vi "Save QOI Image (Path).vi"(8 "error in (no error)":errorcluster, 10 "Image":T1, 11 "Path In":path) -> (0 "error out":errorcluster, 3 "Path Out":path)   [LabVIEW 2020, in "G-Image.lvlib"]
doc: "Saves an image in QOI format to disk."
uses:
  G-Image.lvlib
  <vilib>/picture/picture.llb/imagedata.ctl
  Controls/Image Save Format.ctl
  606af2f9-acf7-4e66-8239-29e2db6da06f.vi
  Private/Debug Path.vi
  Private/Result To Error.vi
  Private/Get Image Data.vi
  Private/ARGB To RGBA.vi
  Private/Depth To Number Channels.vi
  Image Processing/Indexed Color To True Color Image.vi
  <vilib>/Utility/file.llb/Application Directory.vi
  <vilib>/Utility/error.llb/Error Cluster From Error Code.vi
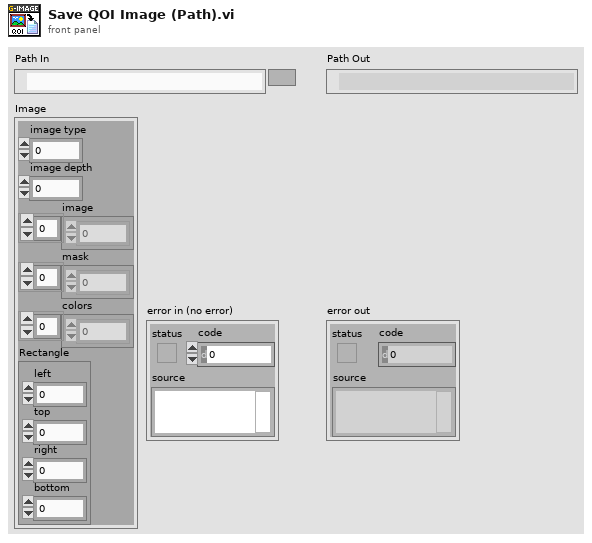
[diagram p1: front panel]
types:
  T1 = typedef "imagedata.ctl" = cluster{"image type":i32, "image depth":i32, "image":u8[], "mask":u8[], "colors":u32[], "Rectangle":cluster{"left":i16, "top":i16, "right":i16, "bottom":i16}}
  T2 = typedef "G-Image.lvlib/Image Save Format.ctl" = enum16{"png", "jpg", "bmp", "gif", "tga", "qoi"}
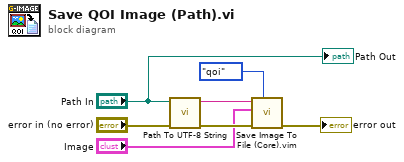
[diagram p0: block diagram]
diagram:
  n1 = call "Path To UTF-8 String.vi"("error in"="error in (no error)", "Path"="Path In") -> ("error out"=w3:errorcluster, "UTF-8 String"=w6:string)  [unwired: 8 in]
  n2 = call "Save Image To File (Core).vim"("Save Format"=Image_Save_Format."qoi", "error in (no error)"=w3, "Picture"="Image", "Path In"=w6) -> ("error out"=→"error out":errorcluster)  [unwired: 6 in, 1 out]
  "Path Out" <- "Path In"
